vi "ChannelHits.vi"(0 "Action":T3(ring)=enum."GetHitsDestructive", 1 "error in":errorcluster, 5 "channel":i32, 7 "Max gethits":i32=3300, 9 "Assert Semaphore":bool=TRUE, 11 "TDCHits":T4[](array[typedef])) -> (3 "Buffer overflow":bool, 4 "Hits":u64[](array[numeric]), 6 "Errors":i64[](array[numeric]), 8 "NumOfHits all channels":i32[][](array[numeric]), 10 "NumOfHits":i32, 12 "Error out":errorcluster, 14 "Amount of hits in ChannelHits global variable":T2(array[cluster]), 15 "NumOfErrors":i32)   [LabVIEW 2016]
uses:
  HPTDC Driver Library Folder/Library files/Typedefs/TDCHit.ctl
  Typedefs/ROB hits.ctl
  HPTDC Driver Library Folder/HPTDC Driver Library.lvlib
panel:
  in  "channel hits":T1[](array[typedef])=[{"ID"=0, "Latest hits"=array[10000 elements], "Newest hit index"=-1, "Max index"=9999, "Amount of hits"=0, "Historical amount of hits"=0}, {"ID"=1, "Latest hits"=array[10000 elements], "Newest hit index"=-1, "Max index"=9999, "Amount of hits"=0, "Historical amount of hits"=0}, {"ID"=2, "Latest hits"=array[10000 elements], "Newest hit index"=-1, "Max index"=9999, "Amount of hits"=0, "Historical amount of hits"=0}, {"ID"=3, "Latest hits"=array[10000 elements], "Newest hit index"=-1, "Max index"=9999, "Amount of hits"=0, "Historical amount of hits"=0}, {"ID"=4, "Latest hits"=array[10000 elements], "Newest hit index"=-1, "Max index"=9999, "Amount of hits"=0, "Historical amount of hits"=0}, {"ID"=5, "Latest hits"=array[10000 elements], "Newest hit index"=-1, "Max index"=9999, "Amount of hits"=0, "Historical amount of hits"=0}, {"ID"=6, "Latest hits"=array[10000 elements], "Newest hit index"=-1, "Max index"=9999, "Amount of hits"=0, "Historical amount of hits"=0}, {"ID"=7, "Latest hits"=array[10000 elements], "Newest hit index"=-1, "Max index"=9999, "Amount of hits"=0, "Historical amount of hits"=0}, {"ID"=8, "Latest hits"=array[10000 elements], "Newest hit index"=-1, "Max index"=9999, "Amount of hits"=0, "Historical amount of hits"=0}, {"ID"=9, "Latest hits"=array[10000 elements], "Newest hit index"=-1, "Max index"=9999, "Amount of hits"=0, "Historical amount of hits"=0}, {"ID"=10, "Latest hits"=array[10000 elements], "Newest hit index"=-1, "Max index"=9999, "Amount of hits"=0, "Historical amount of hits"=0}, {"ID"=11, "Latest hits"=array[10000 elements], "Newest hit index"=-1, "Max index"=9999, "Amount of hits"=0, "Historical amount of hits"=0}, {"ID"=12, "Latest hits"=array[10000 elements], "Newest hit index"=-1, "Max index"=9999, "Amount of hits"=0, "Historical amount of hits"=0}, {"ID"=13, "Latest hits"=array[10000 elements], "Newest hit index"=-1, "Max index"=9999, "Amount of hits"=0, "Historical amount of hits"=0}, {"ID"=14, "Latest hits"=array[10000 elements], "Newest hit index"=-1, "Max index"=9999, "Amount of hits"=0, "Historical amount of hits"=0}, {"ID"=15, "Latest hits"=array[10000 elements], "Newest hit index"=-1, "Max index"=9999, "Amount of hits"=0, "Historical amount of hits"=0}, {"ID"=16, "Latest hits"=array[10000 elements], "Newest hit index"=-1, "Max index"=9999, "Amount of hits"=0, "Historical amount of hits"=0}]
  # "Important: Leave Assert Semaphore unwired normally. Only wire \"false\"\nif you make sure to set and release the semaphore outside of Chnl Hits.\nIt is useful to do so if you want to make many consecutive reads, for example\nof different channels, and also prevent any new data to be written to Chnl\nReads inbetween the reads."
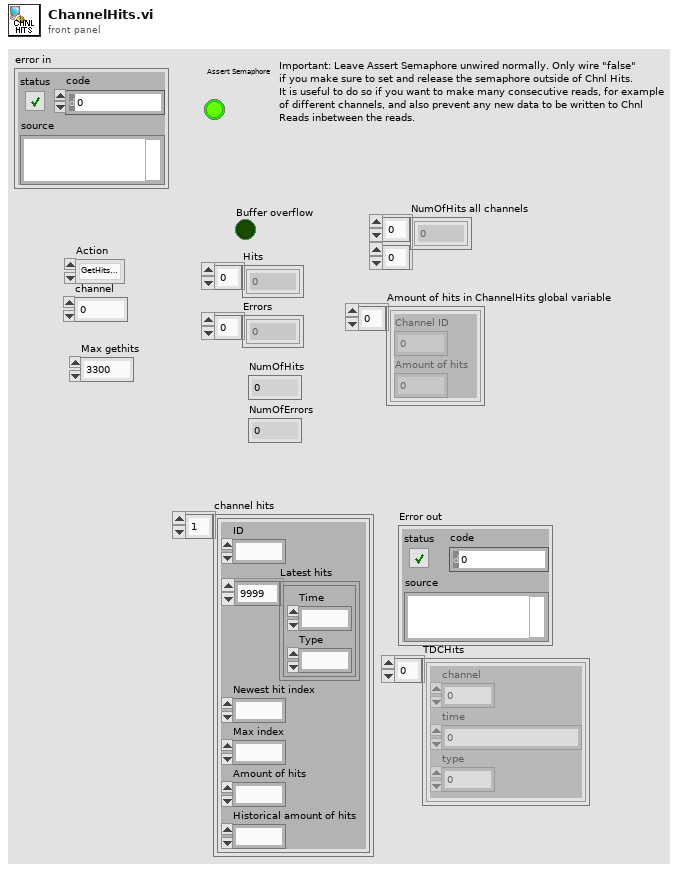
[diagram p1: front panel]
types:
  T1 = typedef "ROB hits.ctl" = cluster{"ID":i32, "Latest hits":cluster{"Time":u64, "Type":i32}[], "Newest hit index":i32, "Max index":i32, "Amount of hits":i32, "Historical amount of hits":u64}
  T2 = cluster{"Channel ID":i32, "Amount of hits":i32}[]
  T3 = enum16{"InsertHits", "GetHits", "GetHitsDestructive", "GetNumOfHits"}
  T4 = typedef "HPTDC Driver Library.lvlib/TDCHit.ctl" = cluster{"channel":u8, "time":u64, "type":u8}
  T5 = typedef "Semaphore RefNum" = refnum<k1>
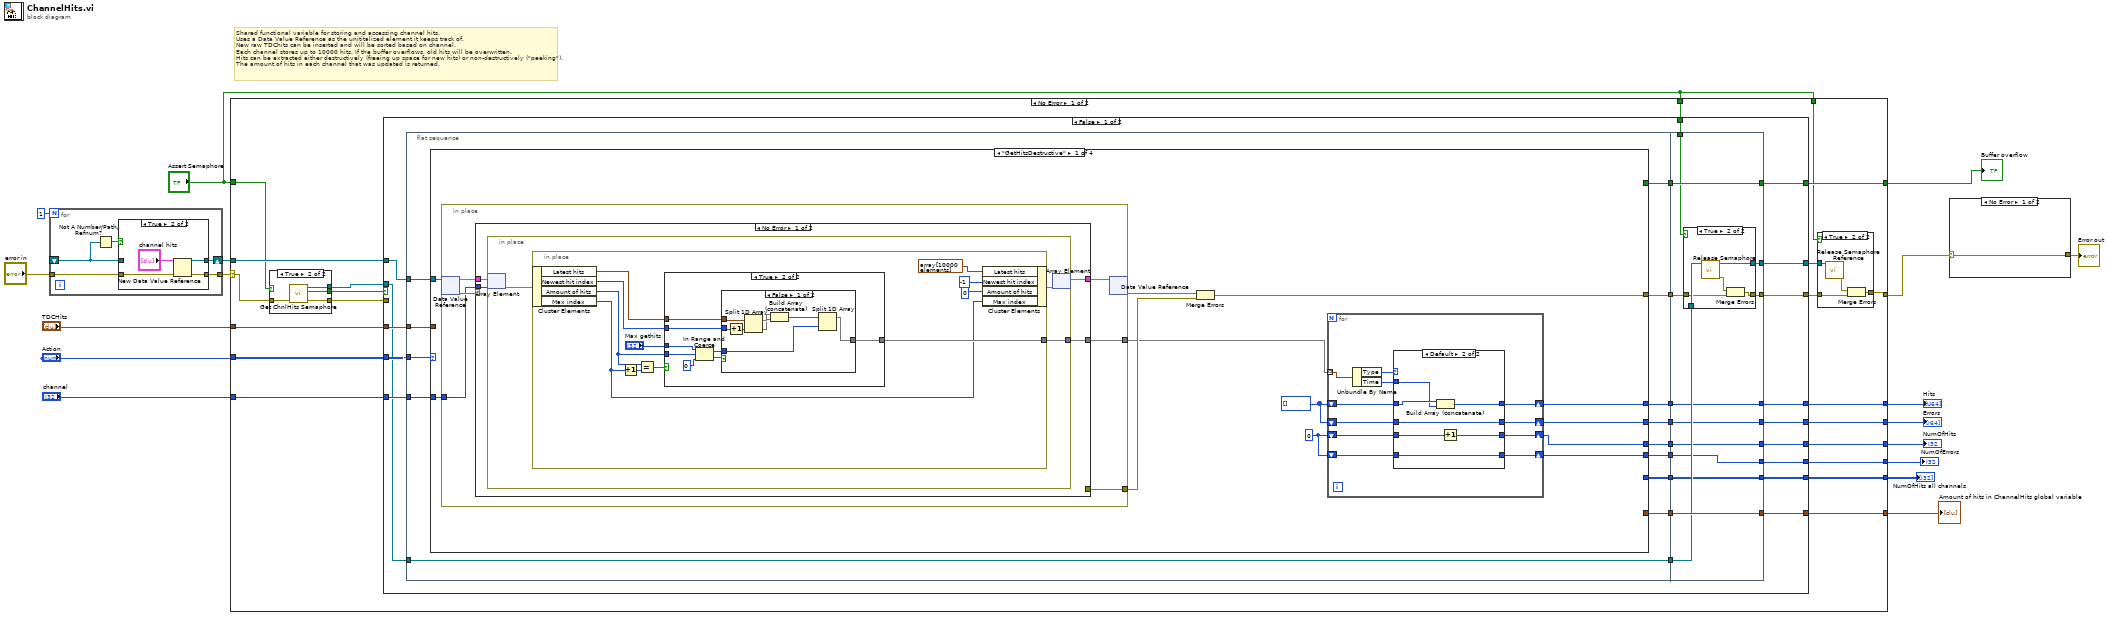
[diagram p0: block diagram]
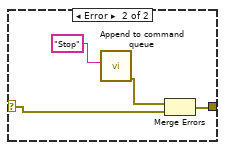
[diagram p2: hidden frame]
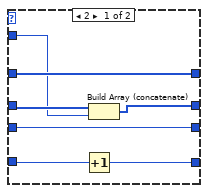
[diagram p5: hidden frame]
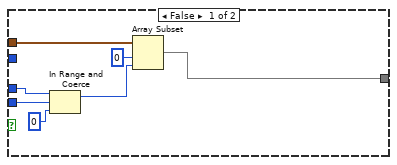
[diagram p6: hidden frame]
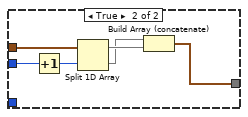
[diagram p7: hidden frame]
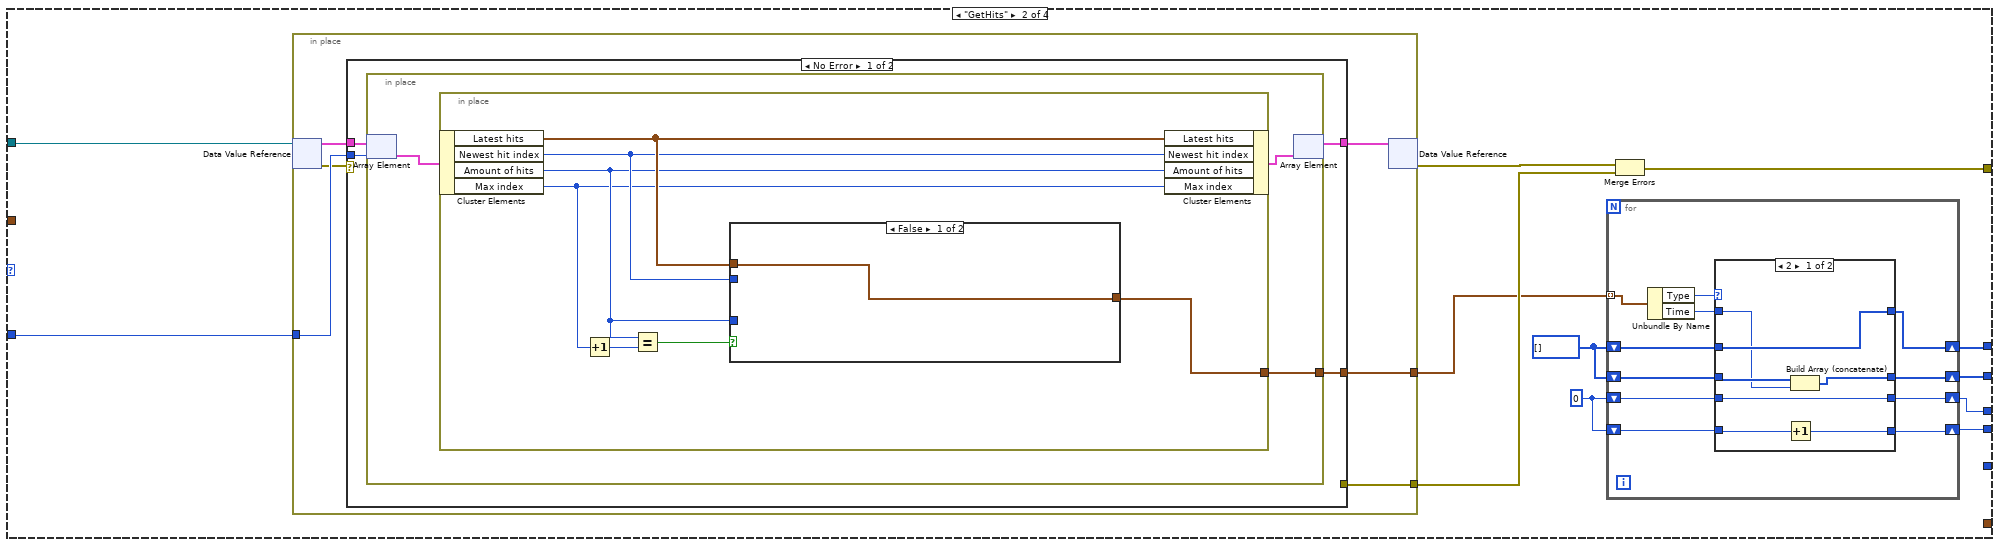
[diagram p9: hidden frame]
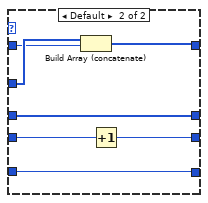
[diagram p10: hidden frame]
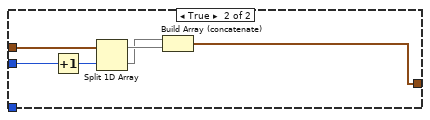
[diagram p11: hidden frame]
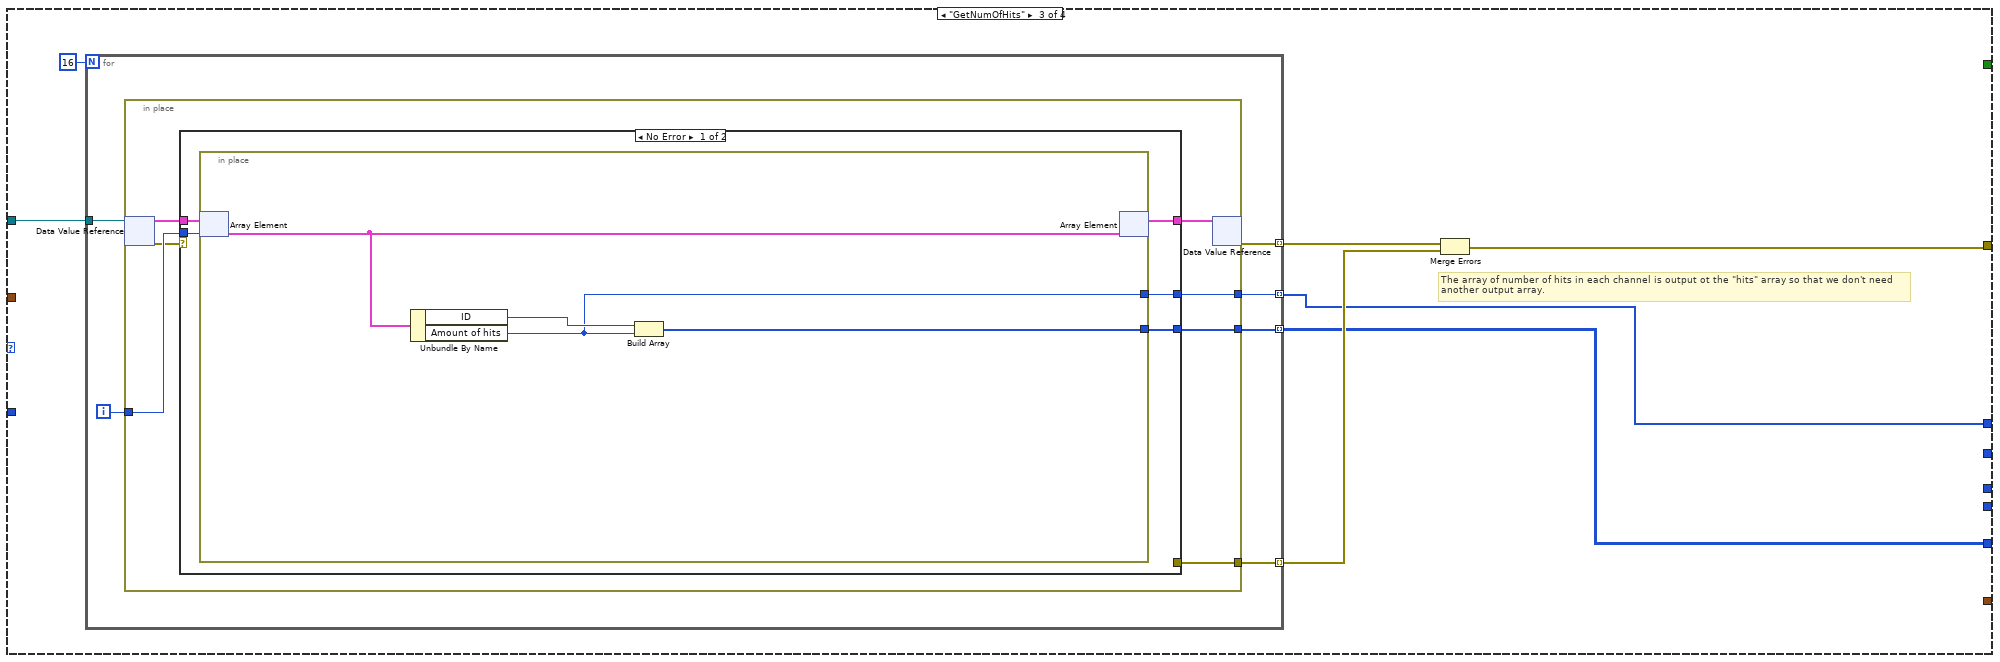
[diagram p13: hidden frame]
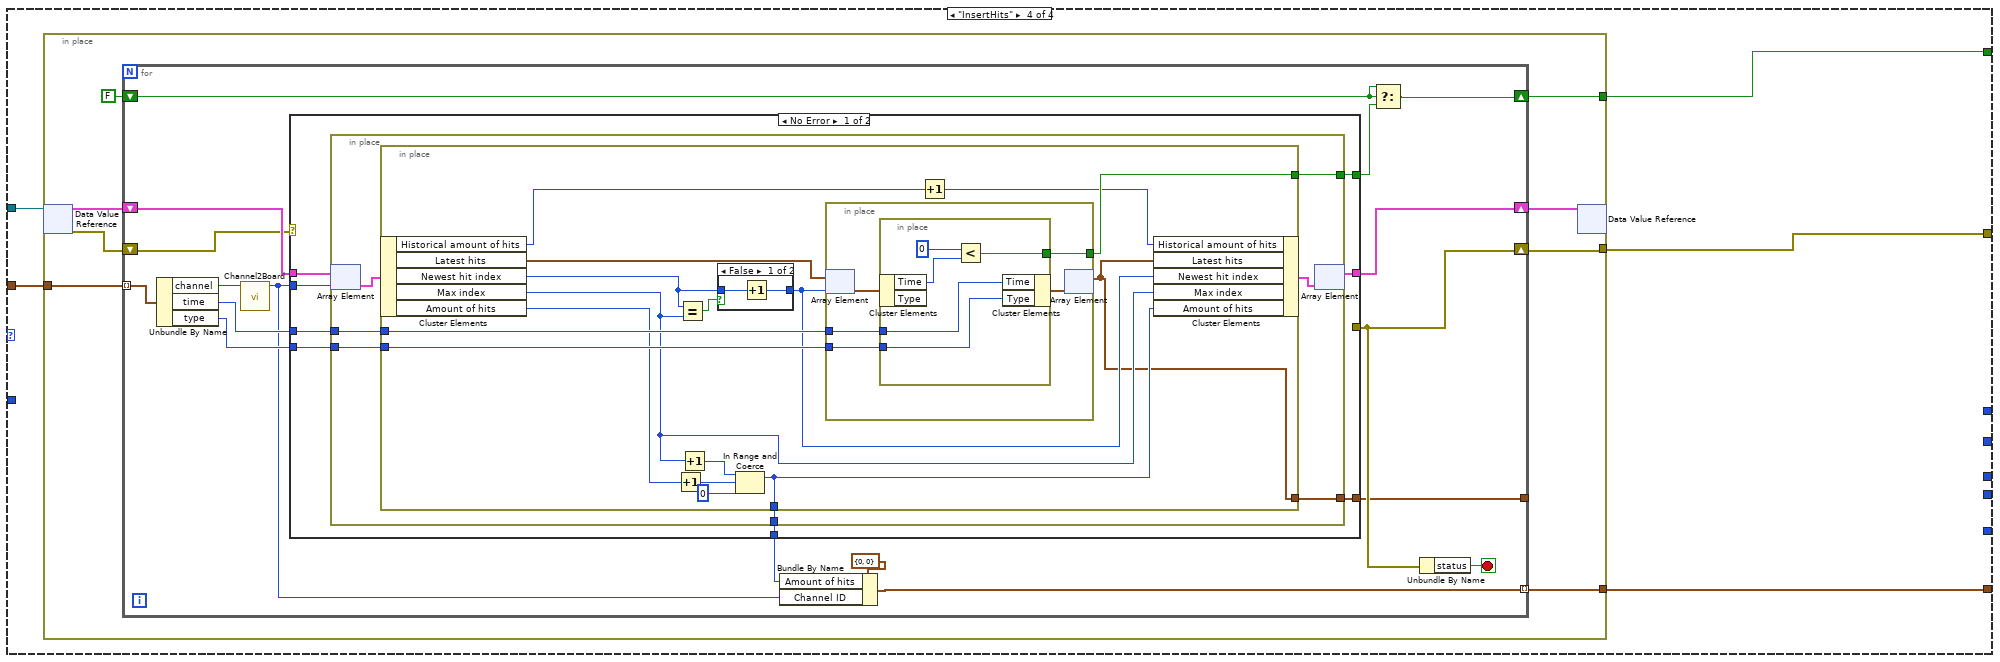
[diagram p15: hidden frame]
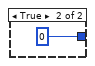
[diagram p16: hidden frame]
diagram:
  # "Shared functional variable for storing and accessing channel hits.\nUses a Data Value Reference as the unititalized element it keeps track of.\nNew raw TDChits can be inserted and will be sorted based on channel.\nEach channel stores up to 10000 hits. If the buffer overflows, old hits will be overwritten.\nHits can be extracted either destructively (freeing up space for new hits) or non-destructively (\"peeking\").\nThe amount of hits in each channel that was updated is returned."
  n1 = for {
    N: 1 -> [_]
    shift-right: [w22] -> w10
    shift-left: _ -> [w20]
    tunnel: "error in" -> [w19]
    tunnel: [w18] -> w9
    n2 = Not A Number/Path/Refnum?(number/path/refnum=w20) -> (NaN/Path/Refnum?=w21:bool)
    n3 = case shown="True" w21 {
      tunnel: [w24 w27] -> w22
      tunnel: w20 -> [w24 _]
      tunnel: w19 -> [w23 w26]
      tunnel: [w23 w25] -> w18
      frame False {
      }
      frame True {
        n4 = New Data Value Reference(data value="channel hits", error in=w26) -> (data value reference=w27:refnum<data-value>, error out=w25:errorcluster)
      }
    }
  }
  n5 = case shown="No Error" w9 {
    selector: w9 -> [w43 w383]
    tunnel: "TDCHits" -> [w49 _]
    tunnel: "Action" -> [w48 _]
    tunnel: "channel" -> [w47 _]
    tunnel: [w46 _] -> w14
    tunnel: [w45 _] -> w13
    tunnel: [w38 w383] -> w8
    tunnel: w10 -> [w44 _]
    tunnel: [w36 _] -> w6
    tunnel: [w35 _] -> w5
    tunnel: [w34 _] -> w4
    tunnel: [w33 _] -> w3
    tunnel: "Assert Semaphore" -> [w30 _]
    tunnel: "Assert Semaphore" -> [w32 _]
    tunnel: "Assert Semaphore" -> [w31 _]
    tunnel: [w29 _] -> w1
    frame No Error {
      n6 = case shown="True" w30 {
        tunnel: w43 -> [w50 w54]
        tunnel: [_ w53] -> w42
        tunnel: [_ w52] -> w41
        tunnel: [w50 w51] -> w37
        frame False {
        }
        frame True {
          n7 = call "Get ChnlHits Semaphore.vi"("error in (no error)"=w54) -> ("error out"=w51:errorcluster, "timed out"=w53:bool, "Refnum out"=w52:T5)  [unwired: 8 in]
        }
      }
      n8 = case shown="False" w42 {
        tunnel: w49 -> [w83 _]
        tunnel: w48 -> [w82 _]
        tunnel: w47 -> [w81 _]
        tunnel: [w80 _] -> w46
        tunnel: [w79 _] -> w45
        tunnel: [w78 w381] -> w39
        tunnel: w44 -> [w77 _]
        tunnel: w41 -> [w73 w382]
        tunnel: [w71 w382] -> w40
        tunnel: w37 -> [_ w381]
        tunnel: [w70 _] -> w36
        tunnel: [w67 _] -> w35
        tunnel: [w65 _] -> w34
        tunnel: [w63 _] -> w33
        tunnel: w32 -> [w62 _]
        tunnel: [w61 _] -> w29
        frame False {
          n9 = flat-sequence {
            tunnel: w83 -> [w96]
            tunnel: w82 -> [w95]
            tunnel: w81 -> [w94]
            tunnel: w77 -> [w90]
            tunnel: [w93] -> w76
            tunnel: [w92] -> w75
            tunnel: [w91] -> w74
            tunnel: w73 -> [w89]
            tunnel: [w89] -> w72
            tunnel: [w88] -> w69
            tunnel: [w87] -> w68
            tunnel: [w86] -> w66
            tunnel: [w85] -> w64
            tunnel: [w84] -> w60
            tunnel: [w369] -> w78
            tunnel: [w372] -> w79
            tunnel: [w373] -> w80
            tunnel: w76 -> [w373]
            tunnel: w75 -> [w372]
            tunnel: w74 -> [w370]
            tunnel: w72 -> [w371]
            tunnel: [w368] -> w71
            tunnel: [w367] -> w70
            tunnel: w69 -> [w367]
            tunnel: w68 -> [w366]
            tunnel: [w366] -> w67
            tunnel: w66 -> [w365]
            tunnel: [w365] -> w65
            tunnel: w64 -> [w364]
            tunnel: [w364] -> w63
            tunnel: w62 -> [w363]
            tunnel: [w362] -> w61
            tunnel: w60 -> [w362]
            frame #0 {
              n10 = case shown="\"GetHitsDestructive\"" w95 {
                tunnel: w96 -> [_ _ _ w290]
                tunnel: w90 -> [w108 w200 w259 w286]
                tunnel: w94 -> [w98 w199 _ _]
                tunnel: [_ _ _ w289] -> w93
                tunnel: [_ _ _ w288] -> w92
                tunnel: [w107 w198 w258 w287] -> w91
                tunnel: [w102 w193 w255 _] -> w88
                tunnel: [w101 w192 _ _] -> w87
                tunnel: [w100 w191 _ _] -> w86
                tunnel: [w99 w190 _ _] -> w85
                tunnel: [_ _ w256 _] -> w84
                frame "GetHitsDestructive" {
                  w104 = 0 ("Time")
                  w103 = u64[] [] ("Array")
                  n11 = in-place {
                    in-place-border: w98 -> [w134]
                    in-place-border: [w138] -> w97
                    in-place-border: [w135] -> w105
                    n12 = in-place-dvr #1(w108) -> (w139:T1[], w136:errorcluster)
                    n13 = case shown="No Error" w136 {
                      selector: w136 -> [_ w188]
                      tunnel: w139 -> [w143 w187]
                      tunnel: w134 -> [w142 _]
                      tunnel: [w141 _] -> w138
                      tunnel: [w140 w187] -> w137
                      tunnel: [_ w188] -> w135
                      frame No Error {
                        n14 = in-place {
                          in-place-border: [w145] -> w141
                          n15 = in-place-array #2(w143, w142) -> (w146:T1)
                          n16 = in-place {
                            in-place-border: [w155] -> w145
                            n17 = in-place-cluster #3(w146) -> ("Latest hits"=w151:cluster{"Time":u64, "Type":i32}[], "Newest hit index"=w153:i32, "Amount of hits"=w154:i32, "Max index"=w152:i32)
                            n18 = Increment(x=w152) -> (x+1=w157:i32)
                            n19 = Equal?(x=w154, y=w157) -> (x = y?=w156:bool)
                            n20 = case shown="True" w156 {
                              tunnel: w151 -> [w163 w172]
                              tunnel: [w162 w170] -> w155
                              tunnel: w154 -> [w161 w168]
                              tunnel: w153 -> [_ w171]
                              tunnel: "Max gethits" -> [w160 w167]
                              frame False {
                                n21 = In Range and Coerce(upper limit=w160, x=w161, lower limit=0) -> (coerced(x)=w159:i32)  [unwired: 1 out]
                                n22 = Array Subset(array=w163, index=0, length=w159) -> (w162:cluster{"Time":u64, "Type":i32}[])
                              }
                              frame True {
                                n23 = In Range and Coerce(upper limit=w167, x=w168, lower limit=0) -> (coerced(x)=w165:i32, In Range?=w166:bool)
                                n24 = case shown="False" w166 {
                                tunnel: w172 -> [w177 w186]
                                tunnel: w171 -> [w176 w184]
                                tunnel: [w173 w181] -> w170
                                tunnel: w165 -> [w174 _]
                                frame False {
                                n25 = Increment(x=w176) -> (x+1=w180:i32)
                                n26 = Split 1D Array(array=w177, index=w180) -> (first subarray=w179:cluster{"Time":u64, "Type":i32}[], second subarray=w178:cluster{"Time":u64, "Type":i32}[])
                                n27 = Build Array (concatenate)(w178, w179) -> (w175:cluster{"Time":u64, "Type":i32}[])
                                n28 = Split 1D Array(array=w175, index=w174) -> (first subarray=w173:cluster{"Time":u64, "Type":i32}[])  [unwired: 1 out]
                                }
                                frame True {
                                n29 = Increment(x=w184) -> (x+1=w185:i32)
                                n30 = Split 1D Array(array=w186, index=w185) -> (first subarray=w183:cluster{"Time":u64, "Type":i32}[], second subarray=w182:cluster{"Time":u64, "Type":i32}[])
                                n31 = Build Array (concatenate)(w182, w183) -> (w181:cluster{"Time":u64, "Type":i32}[])
                                }
                                }
                              }
                            }
                            n32 = in-place-cluster #3("Latest hits"=cluster{"Time":u64, "Type":i32}[] array[10000 elements], "Newest hit index"=-1, "Amount of hits"=0 ("Newest hit index"), "Max index"=w152) -> (w144:T1)
                          }
                          n33 = in-place-array #2(w144) -> (w140:T1[])  [unwired: 1 out]
                        }
                      }
                      frame Error {
                      }
                    }
                    n34 = in-place-dvr #1(w137) -> (w106:errorcluster)  [unwired: 1 out]
                  }
                  n35 = Merge Errors(w106, w105) -> (w107:errorcluster)
                  n36 = for {
                    tunnel: w97 -> [w119] mode=indexing
                    shift-right: [w115] -> w102
                    shift-left: w103 -> [w116]
                    shift-right: [w114] -> w101
                    shift-left: w103 -> [w113]
                    shift-right: [w109] -> w100
                    shift-left: w104 -> [w112]
                    shift-right: [w110] -> w99
                    shift-left: w104 -> [w111]
                    n37 = Unbundle By Name(w119) -> ("Type"=w118:i32, "Time"=w117:u64)
                    n38 = case shown="Default" w118 {
                      tunnel: w117 -> [w124 w132]
                      tunnel: [w126 w131] -> w115
                      tunnel: w116 -> [w126 w133]
                      tunnel: [w123 w130] -> w114
                      tunnel: w113 -> [w125 w130]
                      tunnel: w112 -> [w120 w129]
                      tunnel: w111 -> [w122 w127]
                      tunnel: [w121 w127] -> w110
                      tunnel: [w120 w128] -> w109
                      frame 2 {
                        n39 = Increment(x=w122) -> (x+1=w121:i32)
                        n40 = Build Array (concatenate)(w125, w124) -> (w123:u64[])
                      }
                      frame Default {
                        n41 = Build Array (concatenate)(w133, w132) -> (w131:u64[])
                        n42 = Increment(x=w129) -> (x+1=w128:i32)
                      }
                    }
                  }
                }
                frame "GetHits" {
                  w195 = 0 ("Time")
                  w194 = i64[] [] ("Array")
                  n43 = in-place {
                    in-place-border: w199 -> [w230]
                    in-place-border: [w229] -> w189
                    in-place-border: [w226] -> w196
                    n44 = in-place-dvr #4(w200) -> (w231:T1[], w227:errorcluster)
                    n45 = case shown="No Error" w227 {
                      selector: w227 -> [_ w254]
                      tunnel: w231 -> [w235 w253]
                      tunnel: w230 -> [w234 _]
                      tunnel: [w233 _] -> w229
                      tunnel: [w232 w253] -> w228
                      tunnel: [_ w254] -> w226
                      frame No Error {
                        n46 = in-place {
                          in-place-border: [w237] -> w233
                          n47 = in-place-array #5(w235, w234) -> (w238:T1)
                          n48 = in-place {
                            in-place-border: [w243] -> w237
                            n49 = in-place-cluster #6(w238) -> ("Latest hits"=w242:cluster{"Time":u64, "Type":i32}[], "Newest hit index"=w241:i32, "Amount of hits"=w240:i32, "Max index"=w239:i32)
                            n50 = Increment(x=w239) -> (x+1=w245:i32)
                            n51 = Equal?(x=w240, y=w245) -> (x = y?=w244:bool)
                            n52 = case shown="False" w244 {
                              tunnel: w242 -> [w246 w252]
                              tunnel: [w246 w247] -> w243
                              tunnel: w240 -> [_ _]
                              tunnel: w241 -> [_ w250]
                              frame False {
                              }
                              frame True {
                                n53 = Increment(x=w250) -> (x+1=w251:i32)
                                n54 = Split 1D Array(array=w252, index=w251) -> (first subarray=w249:cluster{"Time":u64, "Type":i32}[], second subarray=w248:cluster{"Time":u64, "Type":i32}[])
                                n55 = Build Array (concatenate)(w248, w249) -> (w247:cluster{"Time":u64, "Type":i32}[])
                              }
                            }
                            n56 = in-place-cluster #6("Latest hits"=w242, "Newest hit index"=w241, "Amount of hits"=w240, "Max index"=w239) -> (w236:T1)
                          }
                          n57 = in-place-array #5(w236) -> (w232:T1[])  [unwired: 1 out]
                        }
                      }
                      frame Error {
                      }
                    }
                    n58 = in-place-dvr #4(w228) -> (w197:errorcluster)  [unwired: 1 out]
                  }
                  n59 = for {
                    tunnel: w189 -> [w211] mode=indexing
                    shift-right: [w207] -> w193
                    shift-left: w194 -> [w208]
                    shift-right: [w206] -> w192
                    shift-left: w194 -> [w205]
                    shift-right: [w201] -> w191
                    shift-left: w195 -> [w204]
                    shift-right: [w202] -> w190
                    shift-left: w195 -> [w203]
                    n60 = Unbundle By Name(w211) -> ("Type"=w210:i32, "Time"=w209:u64)
                    n61 = case shown="2" w210 {
                      tunnel: w209 -> [w216 w224]
                      tunnel: [w218 w223] -> w207
                      tunnel: w208 -> [w218 w225]
                      tunnel: [w215 w222] -> w206
                      tunnel: w205 -> [w217 w222]
                      tunnel: w204 -> [w212 w221]
                      tunnel: w203 -> [w214 w219]
                      tunnel: [w213 w219] -> w202
                      tunnel: [w212 w220] -> w201
                      frame 2 {
                        n62 = Increment(x=w214) -> (x+1=w213:i32)
                        n63 = Build Array (concatenate)(w217, w216) -> (w215:u64[])
                      }
                      frame Default {
                        n64 = Build Array (concatenate)(w225, w224) -> (w223:u64[])
                        n65 = Increment(x=w221) -> (x+1=w220:i32)
                      }
                    }
                  }
                  n66 = Merge Errors(w197, w196) -> (w198:errorcluster)
                }
                frame "GetNumOfHits" {
                  # "The array of number of hits in each channel is output ot the \"hits\" array so that we don't need \nanother output array."
                  n67 = for {
                    N: 16 -> [_]
                    tunnel: [w267] -> w261 mode=indexing
                    tunnel: [w266] -> w260 mode=indexing
                    tunnel: w259 -> [w265]
                    tunnel: [w264] -> w256 mode=indexing
                    tunnel: [w262] -> w255 mode=indexing
                    i -> [w263]
                    n68 = in-place {
                      in-place-border: w263 -> [w273]
                      in-place-border: [w270] -> w266
                      in-place-border: [w269] -> w264
                      in-place-border: [w268] -> w262
                      n69 = in-place-dvr #7(w265) -> (w274:T1[], w271:errorcluster)
                      n70 = case shown="No Error" w271 {
                        selector: w271 -> [_ w285]
                        tunnel: w274 -> [w279 w284]
                        tunnel: w273 -> [w278 _]
                        tunnel: [w277 w284] -> w272
                        tunnel: [_ w285] -> w270
                        tunnel: [w276 _] -> w269
                        tunnel: [w275 _] -> w268
                        frame No Error {
                          n71 = in-place {
                            in-place-border: [w281] -> w276
                            in-place-border: [w280] -> w275
                            n72 = in-place-array #8(w279, w278) -> (w283:T1)
                            n73 = Unbundle By Name(w283) -> ("ID"=w282:i32, "Amount of hits"=w280:i32)
                            n74 = Build Array(w282, w280) -> (w281:i32[])
                            n75 = in-place-array #8(w283) -> (w277:T1[])  [unwired: 1 out]
                          }
                        }
                        frame Error {
                        }
                      }
                      n76 = in-place-dvr #7(w272) -> (w267:errorcluster)  [unwired: 1 out]
                    }
                  }
                  n77 = Merge Errors(w261, w260) -> (w258:errorcluster)
                }
                frame "InsertHits" {
                  n78 = in-place {
                    in-place-border: w290 -> [w298]
                    in-place-border: [w297] -> w289
                    in-place-border: [w296] -> w288
                    in-place-border: [w292] -> w287
                    n79 = in-place-dvr #9(w286) -> (w294:T1[], w293:errorcluster)
                    n80 = for {
                      tunnel: w298 -> [w304] mode=indexing
                      shift-right: [w303] -> w291
                      shift-left: w294 -> [w301]
                      shift-right: [w311] -> w297
                      shift-left: FALSE -> [w312]
                      tunnel: [w307] -> w296 mode=indexing
                      shift-right: [w302] -> w292
                      shift-left: w293 -> [w300]
                      tunnel: [w299] -> _
                      stop <- w306 stop-if-true
                      n81 = Unbundle By Name(w304) -> ("channel"=w313:u8, "time"=w315:u64, "type"=w314:u8)
                      n82 = call "Channel2Board.vi"("channel"=w313) -> ("Numeric"=w305:u8)  [unwired: 10 in]
                      n83 = case shown="No Error" w300 {
                        selector: w300 -> [_ w361]
                        tunnel: w315 -> [w323 _]
                        tunnel: w314 -> [w322 _]
                        tunnel: w305 -> [w321 _]
                        tunnel: w301 -> [w320 w360]
                        tunnel: [w319 w360] -> w303
                        tunnel: [w318 _] -> w310
                        tunnel: [w317 _] -> w308
                        tunnel: [_ w361] -> w302
                        tunnel: [w316 _] -> w299
                        frame No Error {
                          n84 = in-place {
                            in-place-border: w323 -> [w329]
                            in-place-border: w322 -> [w328]
                            in-place-border: [w326] -> w318
                            in-place-border: [w325] -> w317
                            in-place-border: [w324] -> w316
                            n85 = in-place-array #10(w320, w321) -> (w330:T1)
                            n86 = in-place {
                              in-place-border: w329 -> [w346]
                              in-place-border: w328 -> [w345]
                              in-place-border: [w337] -> w326
                              in-place-border: [w335] -> w325
                              in-place-border: [w331] -> w324
                              n87 = in-place-cluster #11(w330) -> ("Historical amount of hits"=w334:u64, "Latest hits"=w332:cluster{"Time":u64, "Type":i32}[], "Newest hit index"=w344:i32, "Max index"=w339:i32, "Amount of hits"=w336:i32)
                              n88 = Increment(x=w336) -> (x+1=w342:i32)
                              n89 = Equal?(x=w344, y=w339) -> (x = y?=w338:bool)
                              n90 = Increment(x=w339) -> (x+1=w340:i32)
                              n91 = case shown="False" w338 {
                                tunnel: [w348 0] -> w343
                                tunnel: w344 -> [w347 _]
                                frame False {
                                n92 = Increment(x=w347) -> (x+1=w348:i32)
                                }
                                frame True {
                                }
                              }
                              n93 = In Range and Coerce(upper limit=w340, x=w342, lower limit=0) -> (coerced(x)=w335:i32)  [unwired: 1 out]
                              n94 = in-place {
                                in-place-border: w346 -> [w354]
                                in-place-border: w345 -> [w353]
                                in-place-border: [w352] -> w337
                                n95 = in-place-array #12(w332, w343) -> (w350:cluster{"Time":u64, "Type":i32})
                                n96 = in-place {
                                in-place-border: w354 -> [w359]
                                in-place-border: w353 -> [w355]
                                in-place-border: [w356] -> w352
                                n97 = in-place-cluster #13(w350) -> ("Time"=w358:u64)  [unwired: 1 out]
                                n98 = Less?(x=i64 0, y=w358) -> (x < y?=w356:bool)
                                n99 = in-place-cluster #13("Time"=w359, "Type"=w355) -> (w351:cluster{"Time":u64, "Type":i32})
                                }
                                n100 = in-place-array #12(w351) -> (w331:cluster{"Time":u64, "Type":i32}[])  [unwired: 1 out]
                              }
                              n101 = Increment(x=w334) -> (x+1=w333:u64)
                              n102 = in-place-cluster #11("Historical amount of hits"=w333, "Latest hits"=w331, "Newest hit index"=w343, "Max index"=w339, "Amount of hits"=w335) -> (w327:T1)
                            }
                            n103 = in-place-array #10(w327) -> (w319:T1[])  [unwired: 1 out]
                          }
                        }
                        frame Error {
                        }
                      }
                      n104 = Bundle By Name(cluster=cluster{"Channel ID":i8, "Amount of hits":i32} {"Channel ID"=0, "Amount of hits"=0}, "Amount of hits"=w308, "Channel ID"=w305) -> (w307:cluster{"Channel ID":i8, "Amount of hits":i32})
                      n105 = Select(t=w312, s=w312, f=w310) -> (s? t:f=w311:bool)
                      n106 = Unbundle By Name(w302) -> ("status"=w306:bool)
                    }
                    n107 = in-place-dvr #9(w291) -> ()  [unwired: 2 out]
                  }
                }
              }
            }
            frame #1 {
              n108 = case shown="True" w363 {
                tunnel: w371 -> [w374 w380]
                tunnel: w370 -> [w375 w379]
                tunnel: [w375 w377] -> w369
                tunnel: [w374 w376] -> w368
                frame False {
                }
                frame True {
                  n109 = call <vilib>:"Release Semaphore.vi"("semaphore"=w380) -> ("error out"=w378:errorcluster, "semaphore out"=w376:T5)  [unwired: 5 in]
                  n110 = Merge Errors(w378, w379) -> (w377:errorcluster)
                }
              }
            }
          }
        }
        frame True {
        }
      }
      n111 = case shown="True" w31 {
        tunnel: w40 -> [_ w59]
        tunnel: w39 -> [w55 w58]
        tunnel: [w55 w57] -> w38
        frame False {
        }
        frame True {
          n112 = call <vilib>:"Release Semaphore Reference.vi"("semaphore"=w59) -> ("error out"=w56:errorcluster)  [unwired: 9 in, 1 out]
          n113 = Merge Errors(w56, w58) -> (w57:errorcluster)
        }
      }
    }
    frame Error {
    }
  }
  "Buffer overflow" <- w14
  "Amount of hits in ChannelHits global variable" <- w13
  "Hits" <- w6
  "Errors" <- w5
  "NumOfHits" <- w4
  "NumOfErrors" <- w3
  "NumOfHits all channels" <- w1
  n114 = case shown="No Error" w8 {
    selector: w8 -> [w384 w385]
    tunnel: [w384 w387] -> w7
    frame No Error {
    }
    frame Error {
      n115 = call "Append to command queue.vi"("Single command"="Stop") -> ("error out"=w386:errorcluster)  [unwired: 10 in]
      n116 = Merge Errors(w386, w385) -> (w387:errorcluster)
    }
  }
  "Error out" <- w7
